vi "诊断标定3 - 副本.vi"(8 "CAN端口":u16(ring), 9 "设备索引号":u16(ring), 10 "CAN卡类型":u32(ring)=21) -> ()   [LabVIEW 2013] (continued)
                        n4271 = control-ref of="一级故障 2"() -> (w6031:refnum<vi>)
                        n4272 = property class="Clust (严格)"(reference=w6031) -> ("Value"=w6053:T10)  [unwired: 1 in, 2 out]
                        n4273 = Unbundle(w6053) -> ("总电压过高"=w6052:dbl, "整组电压不均衡"=w6047:dbl, "SOC过高"=w6040:dbl, "单体电压过高"=w6043:dbl, "总电压过低"=w6051:dbl, "温度过高"=w6050:dbl, "温度过低"=w6049:dbl, "单组电压不均衡"=w6048:dbl, "整组温度不均衡"=w6045:dbl, "单组温度不均衡"=w6046:dbl, "单体电压过低"=w6044:dbl, "充电电流过高"=w6042:dbl, "放电电流过高"=w6041:dbl, "SOC过低"=w6039:dbl, "内阻过大"=w6038:dbl, "极柱温度过高"=w6037:dbl, "SOH过低"=w6036:dbl)
                        n4274 = Build Array(w6052, w6051, w6050, w6049, w6048, w6047, w6046, w6045, w6043, w6044, w6042, w6041, w6040, w6039, w6038, w6037, w6036) -> (w6035:dbl[])
                        n4275 = for {
                          tunnel: w6035 -> [w6055] mode=indexing
                          tunnel: [w6054] -> w6034 mode=indexing
                          n4276 = Format Into String(format string="%#f" ("格式字符串"), w6055) -> (resulting string=w6054:string)  [unwired: 2 in, 1 out]
                        }
                        n4277 = Build Array(string[] ["总电压过高二级", "总电压过低二级", "温度过高二级", "温度过低二级", "单组电压不均衡二级", "整组电压不均衡二级", "单组温度不均衡二级", "整组温度不均衡二级", "单体电压过高二级", "单体电压过低二级", "充电电流过高二级", "放电电流过高二级", "SOC过高二级", "SOC过低二级", "内阻过大二级", "极柱温度过高二级", "SOH过低二级"], w6034) -> (w6032:string[][])
                        n4278 = Transpose 2D Array(2D array=w6032) -> (transposed array=w6030:string[][])
                      }
                      frame #3 {
                        n4279 = control-ref of="一级故障 3"() -> (w6058:refnum<vi>)
                        n4280 = property class="Clust (严格)"(reference=w6058) -> ("Value"=w6080:T10)  [unwired: 1 in, 2 out]
                        n4281 = Unbundle(w6080) -> ("总电压过高"=w6079:dbl, "整组电压不均衡"=w6074:dbl, "SOC过高"=w6067:dbl, "单体电压过高"=w6070:dbl, "总电压过低"=w6078:dbl, "温度过高"=w6077:dbl, "温度过低"=w6076:dbl, "单组电压不均衡"=w6075:dbl, "整组温度不均衡"=w6072:dbl, "单组温度不均衡"=w6073:dbl, "单体电压过低"=w6071:dbl, "充电电流过高"=w6069:dbl, "放电电流过高"=w6068:dbl, "SOC过低"=w6066:dbl, "内阻过大"=w6065:dbl, "极柱温度过高"=w6064:dbl, "SOH过低"=w6063:dbl)
                        n4282 = Build Array(w6079, w6078, w6077, w6076, w6075, w6074, w6073, w6072, w6070, w6071, w6069, w6068, w6067, w6066, w6065, w6064, w6063) -> (w6062:dbl[])
                        n4283 = for {
                          tunnel: w6062 -> [w6082] mode=indexing
                          tunnel: [w6081] -> w6061 mode=indexing
                          n4284 = Format Into String(format string="%#f" ("格式字符串"), w6082) -> (resulting string=w6081:string)  [unwired: 2 in, 1 out]
                        }
                        n4285 = Build Array(string[] ["总电压过高三级", "总电压过低三级", "温度过高三级", "温度过低三级", "单组电压不均衡三级", "整组电压不均衡三级", "单组温度不均衡三级", "整组温度不均衡三级", "单体电压过高三级", "单体电压过低三级", "充电电流过高三级", "放电电流过高三级", "SOC过高三级", "SOC过低三级", "内阻过大三级", "极柱温度过高三级", "SOH过低三级"], w6061) -> (w6059:string[][])
                        n4286 = Transpose 2D Array(2D array=w6059) -> (transposed array=w6057:string[][])
                      }
                      frame #4 {
                        n4287 = control-ref of="加热控制参数"() -> (w6095:refnum<vi>)
                        n4288 = property class="Clust (严格)"(reference=w6095) -> ("Value"=w6094:T11)  [unwired: 1 in, 2 out]
                        n4289 = Unbundle(w6094) -> ("风机开启温度"=w6093:dbl, "风机关闭温度"=w6092:dbl, "加热开启温度"=w6091:dbl, "加热关闭温度"=w6090:dbl, "风机开启温差"=w6089:dbl, "风机关闭温差"=w6088:dbl, "加热关闭温差"=w6084:dbl)
                        n4290 = Build Array(w6093, w6092, w6091, w6090, w6089, w6088, w6084) -> (w6087:dbl[])
                        n4291 = for {
                          tunnel: w6087 -> [w6097] mode=indexing
                          tunnel: [w6096] -> w6085 mode=indexing
                          n4292 = Format Into String(format string="%#f" ("格式字符串"), w6097) -> (resulting string=w6096:string)  [unwired: 2 in, 1 out]
                        }
                      }
                      frame #5 {
                        n4293 = control-ref of="充电控制参数"() -> (w6115:refnum<vi>)
                        n4294 = property class="Clust (严格)"(reference=w6115) -> ("Value"=w6117:T12)  [unwired: 1 in, 2 out]
                        n4295 = Unbundle(w6117) -> ("最大允许单体电压"=w6114:dbl, "最大允许总电压"=w6113:dbl, "最小允许单体电压"=w6112:dbl, "最大允许充电电流"=w6111:dbl, "最小允许充电电流"=w6110:dbl, "最大允许充电温度"=w6109:dbl, "最小允许充电温度"=w6108:dbl, "电流步长"=w6107:dbl)
                        n4296 = Build Array(w6114, w6113, w6112, w6111, w6110, w6109, w6108, w6107) -> (w6116:dbl[])
                        n4297 = for {
                          tunnel: w6116 -> [w6119] mode=indexing
                          tunnel: [w6118] -> w6101 mode=indexing
                          n4298 = Format Into String(format string="%#f" ("格式字符串"), w6119) -> (resulting string=w6118:string)  [unwired: 2 in, 1 out]
                        }
                        n4299 = Insert Into Array(array=w6102, new element=w6101) -> (w6100:string[])  [unwired: 1 in]
                        n4300 = Insert Into Array(array=w6104, new element=string[] ["最大允许单体电压", "最大允许总电压", "最小允许单体电压", "最大允许充电电流", "最小允许充电电流", "最大允许充电温度", "最小允许充电温度", "电流步长"]) -> (w6099:string[])  [unwired: 1 in]
                        n4301 = Build Array(w6099, w6100) -> (w6106:string[][])
                        n4302 = Transpose 2D Array(2D array=w6106) -> (transposed array=w6105:string[][])
                      }
                      frame #6 {
                        n4303 = control-ref of="电池信息"() -> (w6143:refnum<vi>)
                        n4304 = property class="Clust (严格)"(reference=w6143) -> ("Value"=w6146:T13)  [unwired: 1 in, 2 out]
                        n4305 = Unbundle(w6146) -> ("电池串联"=w6142:dbl, "电池并联"=w6141:dbl, "累计放电总安时"=w6139:dbl, "电池包额定容量"=w6138:dbl, "电池包额定能量(kWh)"=w6137:dbl, "电池包额定总电压"=w6136:dbl, "累计充电总安时"=w6140:dbl, "电池充满次数"=w6135:dbl, "电池放空次数"=w6134:dbl, "电池充电次数"=w6133:dbl, "电池生产日期"=w6131:string, "电池厂家"=w6130:string, "电池类型"=w6129:string, "电池包组号"=w6128:string, "电池包产权标识"=w6127:string, "电池应用车型"=w6126:string, "实际容量"=w6121:dbl)
                        n4306 = Build Array(w6131, w6130, w6129, w6128, w6127, w6126) -> (w6125:string[])
                        n4307 = Build Array(w6142, w6141, w6140, w6139, w6138, w6137, w6136, w6135, w6134, w6133, w6121) -> (w6132:dbl[])
                        n4308 = for {
                          tunnel: w6132 -> [w6148] mode=indexing
                          tunnel: [w6147] -> w6124 mode=indexing
                          n4309 = Format Into String(format string="%#f" ("格式字符串"), w6148) -> (resulting string=w6147:string)  [unwired: 2 in, 1 out]
                        }
                        n4310 = Insert Into Array(array=w6125, new element=w6124) -> (w6123:string[])  [unwired: 1 in]
                        n4311 = call <vilib>:"Unset Busy.vi"() -> ()  [unwired: 2 in, 10 out]
                        n4312 = Build Array(string[] ["电池生产日期", "电池厂商", "电池类型", "电池包组号", "电池包产权标识", "电池包应用车型", "电池串联", "电池并联", "累计充电总安时", "累计放电总安时", "电池包额定容量", "电池包额定能量", "电池包额定总电压", "电池充满次数", "电池放空次数", "电池充电次数", "实际容量"], w6123) -> (w6144:string[][])
                        n4313 = Transpose 2D Array(2D array=w6144) -> (transposed array=w6122:string[][])
                      }
                    }
                    n4314 = Insert Into Array(array=w5963, index (col)=2 ("禁用的索引 (列)"), new element #1=w5960, new element #2=w5959, new element #3=w5958, new element #4=w5957, new element #5=w5956) -> (w5961:string[][])  [unwired: 1 in]
                  }
                  frame "从板" {
                    n4315 = local read "从板号"() -> (w6160:u8)
                    n4316 = Number To Decimal String(number=w6160) -> (decimal integer string=w6157:string)  [unwired: 1 out]
                    n4317 = Concatenate Strings("S", w6157) -> (w6158:string)
                    n4318 = Build Array("从板号" ("元素"), w6157) -> (w6155:string[])
                    n4319 = stacked-sequence {
                      seq-local: [string[] ["风机开启温度", "风机关闭温度", "加热开启温度", "加热关闭温度", "风机开启温差", "风机关闭温差", "加热关闭温差"] _ _ _ _ _] -> [_ _ _ w6229 _ _]
                      seq-local: [w6172 _ _ _ _ _] -> [_ _ _ w6225 _ _]
                      seq-local: [_ string[] ["电压过高一级", "电压过低一级", "温度过高一级", "温度过低一级", "电压不均衡一级", "温度不均衡一级", "SOC过低一级"] _ _ _ _] -> [_ _ _ w6228 _ _]
                      seq-local: [_ w6190 _ _ _ _] -> [_ _ _ w6224 _ _]
                      seq-local: [_ _ string[] ["电压过高二级", "电压过低二级", "温度过高二级", "温度过低二级", "电压不均衡二级", "温度不均衡二级", "SOC过低二级"] _ _ _] -> [_ _ _ w6227 _ _]
                      seq-local: [_ _ w6205 _ _ _] -> [_ _ _ w6223 _ _]
                      tunnel: w6155 -> [w6185 _ _ _ _ _]
                      tunnel: [w6174 _ _ _ _ _] -> w6153
                      tunnel: [_ _ _ w6230 _ _] -> w6151
                      tunnel: [_ _ _ _ w6268 _] -> w6150
                      tunnel: [_ _ _ _ _ w6304] -> _
                      frame #0 {
                        w6165 = string[] ["", "", "", "", "", "", "", "", "", "", "  "]
                        n4320 = control-ref of="项目信息 2"() -> (w6184:refnum<vi>)
                        n4321 = property class="Tbl (严格)"(reference=w6184) -> ("Value"=w6162:string[][])  [unwired: 1 in, 2 out]
                        n4322 = control-ref of="加热控制参数"() -> (w6176:refnum<vi>)
                        n4323 = property class="Clust (严格)"(reference=w6176) -> ("Value"=w6183:T11)  [unwired: 1 in, 2 out]
                        n4324 = Unbundle(w6183) -> ("风机开启温度"=w6182:dbl, "风机关闭温度"=w6181:dbl, "加热开启温度"=w6180:dbl, "加热关闭温度"=w6179:dbl, "风机开启温差"=w6178:dbl, "风机关闭温差"=w6177:dbl, "加热关闭温差"=w6171:dbl)
                        n4325 = Build Array(w6182, w6181, w6180, w6179, w6178, w6177, w6171) -> (w6175:dbl[])
                        n4326 = for {
                          tunnel: w6175 -> [w6188] mode=indexing
                          tunnel: [w6187] -> w6172 mode=indexing
                          n4327 = Format Into String(format string="%#f" ("格式字符串"), w6188) -> (resulting string=w6187:string)  [unwired: 2 in, 1 out]
                        }
                        n4328 = Index Array(array=w6162, index (col)=0 ("禁用的索引 (列)")) -> (element=w6169:string[])  [unwired: 1 in]
                        n4329 = Index Array(array=w6162, index (col)=1 ("禁用的索引 (列)")) -> (element=w6168:string[])  [unwired: 1 in]
                        n4330 = Insert Into Array(array=w6169, new element=w6165) -> (w6167:string[])  [unwired: 1 in]
                        n4331 = Insert Into Array(array=w6168, new element=w6165) -> (w6166:string[])  [unwired: 1 in]
                        n4332 = Build Array(w6167, w6166) -> (w6163:string[][])
                        n4333 = Transpose 2D Array(2D array=w6163) -> (transposed array=w6161:string[][])
                        n4334 = Insert Into Array(array=w6161, index (row)=0 ("索引 (行)"), new element=w6185) -> (w6174:string[][])  [unwired: 1 in]
                      }
                      frame #1 {
                        n4335 = control-ref of="一级故障(从板)"() -> (w6201:refnum<vi>)
                        n4336 = property class="Clust (严格)"(reference=w6201) -> ("Value"=w6200:T15)  [unwired: 1 in, 2 out]
                        n4337 = Unbundle(w6200) -> ("电压过高"=w6199:dbl, "电压过低"=w6198:dbl, "温度过高"=w6197:dbl, "温度过低"=w6196:dbl, "电压不均衡(V)"=w6195:dbl, "温度不均衡"=w6194:dbl, "SOC过低"=w6193:dbl)
                        n4338 = Build Array(w6199, w6198, w6197, w6196, w6195, w6194, w6193) -> (w6192:dbl[])
                        n4339 = for {
                          tunnel: w6192 -> [w6203] mode=indexing
                          tunnel: [w6202] -> w6190 mode=indexing
                          n4340 = Format Into String(format string="%#f" ("格式字符串"), w6203) -> (resulting string=w6202:string)  [unwired: 2 in, 1 out]
                        }
                      }
                      frame #2 {
                        n4341 = control-ref of="二级故障(从板)"() -> (w6207:refnum<vi>)
                        n4342 = property class="Clust (严格)"(reference=w6207) -> ("Value"=w6216:T15)  [unwired: 1 in, 2 out]
                        n4343 = Unbundle(w6216) -> ("电压过高"=w6215:dbl, "电压过低"=w6214:dbl, "温度过高"=w6213:dbl, "温度过低"=w6212:dbl, "电压不均衡(V)"=w6211:dbl, "温度不均衡"=w6210:dbl, "SOC过低"=w6209:dbl)
                        n4344 = Build Array(w6215, w6214, w6213, w6212, w6211, w6210, w6209) -> (w6208:dbl[])
                        n4345 = for {
                          tunnel: w6208 -> [w6218] mode=indexing
                          tunnel: [w6217] -> w6205 mode=indexing
                          n4346 = Format Into String(format string="%#f" ("格式字符串"), w6218) -> (resulting string=w6217:string)  [unwired: 2 in, 1 out]
                        }
                      }
                      frame #3 {
                        n4347 = control-ref of="三级故障(从板)"() -> (w6231:refnum<vi>)
                        n4348 = property class="Clust (严格)"(reference=w6231) -> ("Value"=w6241:T15)  [unwired: 1 in, 2 out]
                        n4349 = Unbundle(w6241) -> ("电压过高"=w6240:dbl, "电压过低"=w6239:dbl, "温度过高"=w6238:dbl, "温度过低"=w6237:dbl, "电压不均衡(V)"=w6236:dbl, "温度不均衡"=w6235:dbl, "SOC过低"=w6234:dbl)
                        n4350 = Build Array(w6240, w6239, w6238, w6237, w6236, w6235, w6234) -> (w6233:dbl[])
                        n4351 = for {
                          tunnel: w6233 -> [w6243] mode=indexing
                          tunnel: [w6242] -> w6222 mode=indexing
                          n4352 = Format Into String(format string="%#f" ("格式字符串"), w6243) -> (resulting string=w6242:string)  [unwired: 2 in, 1 out]
                        }
                        n4353 = Insert Into Array(array=w6229, new element #1=w6228, new element #2=w6227, new element #3=string[] ["电压过高三级", "电压过低三级", "温度过高三级", "温度过低三级", "电压不均衡三级", "温度不均衡三级", "SOC过低三级"]) -> (w6220:string[])  [unwired: 1 in]
                        n4354 = Insert Into Array(array=w6225, new element #1=w6224, new element #2=w6223, new element #3=w6222) -> (w6221:string[])  [unwired: 1 in]
                        n4355 = Build Array(w6220, w6221) -> (w6232:string[][])
                        n4356 = Transpose 2D Array(2D array=w6232) -> (transposed array=w6230:string[][])
                      }
                      frame #4 {
                        n4357 = control-ref of="快换(从板)"() -> (w6267:refnum<vi>)
                        n4358 = property class="Clust (严格)"(reference=w6267) -> ("Value"=w6280:T16)  [unwired: 1 in, 2 out]
                        n4359 = Unbundle(w6280) -> ("串联数"=w6279:dbl, "并联数"=w6278:dbl, "电池厂家"=w6277:dbl, "电池类型"=w6276:dbl, "额定能量"=w6275:dbl, "额定容量"=w6274:dbl, "实际容量"=w6273:dbl, "额定总压"=w6266:dbl, "产权标识"=w6265:dbl, "应用车型"=w6264:dbl, "电池包组号"=w6263:dbl, "SOC"=w6261:dbl, "充电总安时"=w6260:dbl, "放电总安时"=w6259:dbl, "放空次数"=w6258:dbl, "充满次数"=w6257:dbl, "充电次数"=w6256:dbl, "车牌号"=w6246:string, "生产日期"=w6245:string, "最大允许单体电压"=w6255:dbl, "最大允许总电压"=w6254:dbl, "最大允许温度"=w6253:dbl, "最小允许温度"=w6252:dbl, "最大允许充电电流"=w6251:dbl, "最小允许充电电流"=w6250:dbl, "最小允许单体电压"=w6249:dbl, "电流步长"=w6248:dbl, "电池包序号"=w6247:dbl)
                        n4360 = Build Array(w6279, w6278, w6277, w6276, w6275, w6274, w6273, w6266, w6265, w6264, w6263, w6261, w6260, w6259, w6258, w6257, w6256, w6255, w6254, w6253, w6252, w6251, w6250, w6249, w6248, w6247) -> (w6272:dbl[])
                        n4361 = for {
                          tunnel: w6272 -> [w6282] mode=indexing
                          tunnel: [w6281] -> w6270 mode=indexing
                          n4362 = Format Into String(format string="%#f" ("格式字符串"), w6282) -> (resulting string=w6281:string)  [unwired: 2 in, 1 out]
                        }
                        n4363 = Insert Into Array(array=w6270, new element #1=w6246, new element #2=w6245) -> (w6262:string[])  [unwired: 1 in]
                        n4364 = call <vilib>:"Unset Busy.vi"() -> ()  [unwired: 2 in, 10 out]
                        n4365 = Build Array(string[] ["电池串联数", "电池并联数", "电池厂家", "额定能量", "额定容量", "实际容量", "额定总压", "产权标识", "应用车型", "电池包组号", "SOC", "充电总安时", "放电总安时", "放空次数", "充满次数", "充电次数", "最大允许单体电压", "最大允许总电压", "最大允许温度", "最小允许温度", "最大允许充电电流", "最小允许充电电流", "最小允许单体电压", "电流步长", "电池包序号"], w6262) -> (w6271:string[][])
                        n4366 = Transpose 2D Array(2D array=w6271) -> (transposed array=w6268:string[][])
                      }
                      frame #5 {
                        n4367 = local read "均衡参数"() -> (w6303:T17)
                        n4368 = Unbundle(w6303) -> ("充电结束电压(90%)"=w6295:sgl, "充电结束电压(91%)"=w6294:sgl, "充电结束电压(92%)"=w6293:sgl, "充电结束电压(93%)"=w6292:sgl, "充电结束电压(94%)"=w6291:sgl, "均衡计算-电压高阀值1级"=w6302:sgl, "均衡计算-电压高阀值2级"=w6301:sgl, "均衡计算-电压低阀值1级"=w6300:sgl, "均衡计算-电压低阀值2级"=w6299:sgl, "均衡计算-最低电压阀值"=w6298:sgl, "均衡停止-最低电压阀值"=w6297:sgl, "均衡计算-电压极差阀值"=w6296:sgl, "充电结束电压(95%)"=w6290:sgl, "充电结束电压(96%)"=w6289:sgl, "充电结束电压(97%)"=w6288:sgl, "充电结束电压(98%)"=w6287:sgl, "充电结束电压(99%)"=w6286:sgl, "充电结束电压(100%)"=w6285:sgl)
                        n4369 = Build Array(w6302, w6301, w6300, w6299, w6298, w6297, w6296, w6295, w6294, w6293, w6292, w6291, w6290, w6289, w6288, w6287, w6286, w6285) -> (w6307:sgl[])
                        n4370 = for {
                          tunnel: w6307 -> [w6309] mode=indexing
                          tunnel: [w6308] -> w6284 mode=indexing
                          n4371 = Format Into String(format string="%#f" ("格式字符串"), w6309) -> (resulting string=w6308:string)  [unwired: 2 in, 1 out]
                        }
                        n4372 = call <vilib>:"Unset Busy.vi"() -> ()  [unwired: 2 in, 10 out]
                        n4373 = Build Array(string[] ["均衡计算-电压高阀值1级", "均衡计算-电压高阀值2级", "均衡计算-电压低阀值1级", "均衡计算-电压低阀值2级", "均衡计算-最低电压阀值", "均衡停止-最低电压阀值", "均衡计算-电压极差阀值", "充电结束电压(90%)", "充电结束电压(91%)", "充电结束电压(92%)", "充电结束电压(93%)", "充电结束电压(94%)", "充电结束电压(95%)", "充电结束电压(96%)", "充电结束电压(97%)", "充电结束电压(98%)", "充电结束电压(99%)", "充电结束电压(100%)"], w6284) -> (w6306:string[][])
                        n4374 = Transpose 2D Array(2D array=w6306) -> (transposed array=w6304:string[][])
                      }
                    }
                    n4375 = Insert Into Array(array=w6153, index (col)=2 ("禁用的索引 (列)"), new element #1=w6151, new element #2=w6150) -> (w6152:string[][])  [unwired: 1 in]
                  }
                }
                n4376 = call "当前时间解析-8.6.vi"() -> ("名称格式时间"=w5944:string)  [unwired: 1 in, 18 out]
                n4377 = Concatenate Strings(w5944, w5943, ".txt" ("字符串")) -> (w5941:string)
                n4378 = call "自适应屏幕分辨率.vi"() -> ()  [unwired: 16 in]
                n4379 = call "文件对话框2"("prompt"="选择保存的路径", "default name"=w5941, "pattern (all files)"="*.txt") -> ("selected path"=w5939:path, "cancelled"=w5938:bool, "error out"=w5937:errorcluster)  [unwired: 9 in, 1 out]
                n4380 = call <vilib>:"Clear Errors.vi"("error in (no error)"=w5937) -> ()  [unwired: 6 in, 1 out]
                n4381 = case shown="假" w5938 {
                  tunnel: w5945 -> [w5950 _]
                  tunnel: w5939 -> [w5946 _]
                  frame False {
                    n4382 = call-poly <vilib>:"Write To Spreadsheet File.vi"("append to file? (new file:F)"=FALSE, "2D data"=w5950, "file path (dialog if empty)"=w5946) -> ("new file path (Not A Path if cancelled)"=w5948:path)  [unwired: 3 in, 2 out]
                    n4383 = Path To String(path=w5948) -> (string=w5947:string)
                    n4384 = stacked-sequence {
                      tunnel: w5947 -> [w5953]
                      frame #0 {
                        n4385 = Concatenate Strings("保存完成,路径为:" ("字符串"), w5953) -> (w5954:string)
                        n4386 = One Button Dialog(message=w5954, button name ("OK")="是" ("按钮名称（“确定”）")) -> ()  [unwired: 1 out]
                      }
                    }
                  }
                  frame True {
                  }
                }
              }
              frame Disabled {
                n4387 = stacked-sequence {
                  seq-local: [w6324] -> [_]
                  frame #0 {
                    n4388 = local read "项目信息"() -> (w6326:string[][])
                    n4389 = local read "项目信息2"() -> (w6323:T9)
                    n4390 = Array Subset(array=w6326, index (row)=0 ("索引"), index (col)=0 ("索引"), length (col)=2 ("索引")) -> (w6329:string[][])  [unwired: 1 in]
                    n4391 = local read "一级故障"() -> ()  [unwired: 1 out]
                    n4392 = local read "从板个数"() -> (w6324:dbl)
                    n4393 = Unbundle(w6323) -> ("电池额定容量(A)"=w6322:dbl, "电池实际容量(A)"=w6321:dbl, "车架(牌)号"=w6315:string, "配置文件版本"=w6314:string, "SOH(%)"=w6319:dbl, "SOC(%)"=w6320:dbl, "产品编号"=w6316:string)  [unwired: 2 out]
                    n4394 = Index Array(array=w6329, index (col) #1=1 ("禁用的索引 (列)"), index (col) #2=0 ("索引 (列)")) -> (element #1=w6313:string[], element #2=w6312:string[])  [unwired: 2 in]
                    n4395 = Build Array(w6322, w6321, w6320, w6319) -> (w6318:dbl[])
                    n4396 = Number To Decimal String(number=w6324) -> ()  [unwired: 1 in, 1 out]
                    n4397 = for {
                      tunnel: w6318 -> [w6334] mode=indexing
                      tunnel: [w6333] -> w6317 mode=indexing
                      n4398 = Format Into String(format string="%#f" ("格式字符串"), w6334) -> (resulting string=w6333:string)  [unwired: 2 in, 1 out]
                    }
                    n4399 = Insert Into Array(array=w6317, new element #1=w6316, new element #2=w6315, new element #3=w6314, new element #4=w6313) -> ()  [unwired: 1 in, 1 out]
                    n4400 = Insert Into Array(array=string[] ["电池额定容量", "电池实际容量", "SOC", "SOH", "产品编号", "车架(牌)号", "配置文件版本"], new element=w6312) -> ()  [unwired: 1 in, 1 out]
                  }
                }
              }
            }
          }
          frame "读配置文件" {
            n4401 = local read "主从选择"() -> (w6347:enum32{"主板", "从板"})
            n4402 = case shown="\"主板\", 默认" w6347 {
              tunnel: ["M" ("pattern (all files)") "S" ("pattern (all files)")] -> _
              tunnel: ["主板" ("pattern (all files)") "从板" ("pattern (all files)")] -> w6346
              frame "主板", Default {
              }
              frame "从板" {
              }
            }
            n4403 = case shown="真" "布尔" {
              tunnel: [w6749 w6754] -> w6339
              tunnel: [FALSE ("cancelled") w6753] -> _
              tunnel: w6346 -> [_ w6752]
              frame False {
                n4404 = local read "路径"() -> (w6749:path)
              }
              frame True {
                n4405 = global read "配置文件全局.vi" "诊断标定读取地址"() -> (w6750:path)
                n4406 = call "文件对话框"("start path"=w6750, "prompt"="选择要读取的配置文件", "button label"=w6752) -> ("selected path"=w6754:path, "cancelled"=w6753:bool, "error out"=w6751:errorcluster)  [unwired: 4 in, 6 out]
                n4407 = call <vilib>:"Clear Errors.vi"("error in (no error)"=w6751) -> ()  [unwired: 7 out]
              }
            }
            n4408 = Strip Path(path=w6339) -> (stripped path=w6335:path, name=w6343:string)
            n4409 = Match Pattern(string=w6343, regular expression=".ini" ("正则表达式")) -> (offset past match=w6341:i32)  [unwired: 1 in, 3 out]
            n4410 = control-ref of="结果"() -> (w6345:refnum<vi>)
            n4411 = global write "配置文件全局.vi" "诊断标定读取地址"(w6335) -> ()
            n4412 = Not Equal?(x=w6341, y=-1) -> (x != y?=w6336:bool)
            n4413 = case shown="真" w6336 {
              tunnel: w6339 -> [_ w6356]
              tunnel: [_ w6365] -> w6337
              frame False {
              }
              frame True {
                w6368 = "MD5码" ("key")
                w6369 = "总信息" ("section")
                n4414 = Strip Path(path=w6356) -> (stripped path=w6354:path, name=w6353:string)
                n4415 = Match Pattern(string=w6353, regular expression=".ini" ("正则表达式")) -> (before substring=w6350:string, match substring=w6351:string)  [unwired: 1 in, 2 out]
                n4416 = Concatenate Strings(w6350, "-rc" ("字符串"), w6351) -> (w6349:string)
                n4417 = Build Path(base path=w6354, name or relative path=w6349) -> (appended path=w6355:path)
                n4418 = Copy(10:w6355, 11:w6356) -> (3:w6360:path)  [unwired: 3 in, 2 out]
                n4419 = call <vilib>:"Open Config Data.vi"("create file if necessary (T)"=FALSE, "configuration file path"=w6360) -> ("refnum"=w6371:T25)  [unwired: 7 in, 2 out]
                n4420 = call-poly <vilib>:"Read Key.vi"("section"=w6369, "key"=w6368, "refnum"=w6371) -> ("value"=w6366:string, "refnum out"=w6370:T25)  [unwired: 5 in, 2 out]
                n4421 = call-poly <vilib>:"Write Key.vi"("section"=w6369, "value"=w6368, "key"=w6368, "refnum"=w6370) -> ("error out"=w6364:errorcluster, "found?"=w6363:bool, "refnum out"=w6362:T25)  [unwired: 5 in]
                n4422 = call <vilib>:"Close Config Data.vi"("error in (no error)"=w6364, "write file if changed (T)"=w6363, "refnum"=w6362) -> ("error out"=w6361:errorcluster, "file path"=w6358:path)  [unwired: 7 in]
                n4423 = call <vilib>:"MD5Checksum File.vi"("error in (no error)"=w6361, "Path"=w6358) -> ("error out"=w6359:errorcluster, "MD5 message-digest"=w6367:string)  [unwired: 8 in]
                n4424 = Equal?(x=w6367, y=w6366) -> (x = y?=w6365:bool)
                n4425 = Delete(path (use dialog)=w6358, error in=w6359) -> (error out=w6357:errorcluster)  [unwired: 3 in, 2 out]
                n4426 = call <vilib>:"Clear Errors.vi"("error in (no error)"=w6357) -> ()  [unwired: 6 in, 1 out]
              }
            }
            n4427 = And(x=w6336, y=w6337) -> (x .and. y?=w6338:bool)
            n4428 = case shown="真" w6338 {
              tunnel: w6339 -> [_ w6389]
              tunnel: w6345 -> [w6375 w6388]
              tunnel: w6337 -> [w6374 _]
              tunnel: w6336 -> [w6373 _]
              frame False {
                n4429 = stacked-sequence {
                  tunnel: w6373 -> [w6377 _]
                  tunnel: w6375 -> [w6376 w6383]
                  tunnel: w6374 -> [_ w6382]
                  frame #0 {
                    n4430 = case shown="假" w6377 {
                      tunnel: w6376 -> [w6379 _]
                      frame False {
                        n4431 = Build Array("文件格式错误") -> (w6380:string[])
                        n4432 = call "表格编辑.vi"("新元素/子数组"=w6380, "活动单元格:单元格背景色"=u32 16711680, "MCListbox引用句柄"=w6379) -> ()  [unwired: 9 out]
                      }
                      frame True {
                      }
                    }
                  }
                  frame #1 {
                    n4433 = case shown="假" w6382 {
                      tunnel: w6383 -> [w6385 _]
                      frame False {
                        n4434 = Build Array("文件MD5码验证错误") -> (w6386:string[])
                        n4435 = call "表格编辑.vi"("新元素/子数组"=w6386, "活动单元格:单元格背景色"=u32 16711680, "MCListbox引用句柄"=w6385) -> ()  [unwired: 9 out]
                      }
                      frame True {
                      }
                    }
                  }
                }
                n4436 = call <vilib>:"Unset Busy.vi"() -> ()  [unwired: 11 in, 1 out]
              }
              frame True {
                n4437 = stacked-sequence {
                  seq-local: [w6394 _ _ _] -> [_ w6622 w6716 _]
                  seq-local: [w6392 _ _ _] -> [_ w6600 _ _]
                  tunnel: w6389 -> [w6390 _ _ _]
                  tunnel: w6388 -> [w6407 _ _ w6743]
                  frame #0 {
                    w6391 = string[][] []
                    w6404 = "总信息" ("section")
                    n4438 = local write "路径"(w6390) -> ()
                    n4439 = call <vilib>:"Open Config Data.vi"("create file if necessary (T)"=FALSE, "configuration file path"=w6390) -> ("error out"=w6395:errorcluster, "refnum"=w6394:T25)  [unwired: 7 in, 1 out]
                    n4440 = call <vilib>:"Get Key Names.vi"("section"=w6404, "error in (no error)"=w6395, "refnum"=w6394) -> ("key names"=w6403:string[], "refnum out"=w6405:T25)  [unwired: 5 in, 2 out]
                    n4441 = for {
                      tunnel: w6405 -> [w6411]
                      tunnel: w6404 -> [w6410]
                      tunnel: w6403 -> [w6409] mode=indexing
                      tunnel: [w6408] -> w6400 mode=indexing
                      n4442 = call-poly <vilib>:"Read Key.vi"("section"=w6410, "key"=w6409, "refnum"=w6411) -> ("value"=w6408:string)  [unwired: 5 in, 3 out]
                    }
                    n4443 = Index Array(array=w6400) -> (element #1=w6393:string, element #2=w6398:string)  [unwired: 2 in]
                    n4444 = Decimal String To Number(string=w6393) -> (number=w6392:i32)  [unwired: 2 in, 1 out]
                    n4445 = Concatenate Strings("正在读取" ("字符串"), w6398, "的配置文件" ("字符串")) -> (w6396:string)
                    n4446 = Build Array(w6396) -> (w6401:string[])
                    n4447 = call "表格编辑.vi"("新元素/子数组"=w6401, "活动单元格:单元格背景色"=u32 6618880, "MCListbox引用句柄"=w6407) -> ()  [unwired: 9 out]
                    n4448 = local write "项目信息"(w6391) -> ()
                    n4449 = local write "项目信息 2"(w6391) -> ()
                  }
                  frame #1 {
                    w6582 = 20 ("长度")
                    w6623 = "主板" ("section")
                    n4450 = call <vilib>:"Get Key Names.vi"("section"=w6623, "refnum"=w6622) -> ("key names"=w6424:string[], "refnum out"=w6624:T25)  [unwired: 6 in, 2 out]
                    n4451 = for {
                      tunnel: w6624 -> [w6636]
                      tunnel: w6623 -> [w6635]
                      tunnel: w6424 -> [w6634] mode=indexing
                      tunnel: [w6633] -> w6423 mode=indexing
                      n4452 = call-poly <vilib>:"Read Key.vi"("section"=w6635, "key"=w6634, "refnum"=w6636) -> ("value"=w6633:string)  [unwired: 5 in, 3 out]
                    }
                    n4453 = Search 1D Array(1D array=w6424, element="总电压过高一级" ("元素"), start index (0)=0 ("开始索引(0)")) -> (index of element=w6504:i32)
                    n4454 = Search 1D Array(1D array=w6424, element="风机开启温度" ("元素"), start index (0)=w6504) -> (index of element=w6495:i32)
                    n4455 = Search 1D Array(1D array=w6424, element="电池串联" ("元素"), start index (0)=w6495) -> (index of element=w6493:i32)
                    n4456 = Decrement(x=w6504) -> (x-1=w6621:i32)
                    n4457 = Array Subset(array=w6424, index=1 ("索引"), length=w6621) -> (w6469:string[])
                    n4458 = Array Subset(array=w6423, index=1 ("索引"), length=w6621) -> (w6466:string[])
                    n4459 = Delete From Array(array=w6466, length=7 ("长度"), index=0 ("索引")) -> (deleted portion=w6463:string[], array with subset deleted=w6413:string[])
                    n4460 = Delete From Array(array=w6469, length=7 ("长度"), index=0 ("索引")) -> (array with subset deleted=w6422:string[])  [unwired: 1 out]
                    n4461 = Search 1D Array(1D array=w6424, element="分流器型号" ("元素")) -> (index of element=w6427:i32)  [unwired: 1 in]
                    n4462 = Index Array(array=w6423, index=0 ("索引")) -> (element=w6597:string)
                    n4463 = Decimal String To Number(string=w6597) -> (number=w6414:i32)  [unwired: 2 in, 1 out]
                    n4464 = Search 1D Array(1D array=w6422, element="主板电池节数" ("元素")) -> (index of element=w6588:i32)  [unwired: 1 in]
                    n4465 = Search 1D Array(1D array=w6422, element="主板温度起始值" ("元素")) -> (index of element=w6585:i32)  [unwired: 1 in]
                    n4466 = Search 1D Array(1D array=w6422, element="第一个保险通道" ("元素")) -> (index of element=w6584:i32)  [unwired: 1 in]
                    n4467 = Search 1D Array(1D array=w6422, element="主板温度个数" ("元素")) -> (index of element=w6586:i32)  [unwired: 1 in]
                    n4468 = Search 1D Array(1D array=w6422, element="主板电压起始值" ("元素")) -> (index of element=w6587:i32)  [unwired: 1 in]
                    n4469 = Search 1D Array(1D array=w6422, element="第1通道电压个数" ("元素")) -> (index of element=w6583:i32)  [unwired: 1 in]
                    n4470 = Index Array(array=w6423, index=w6427) -> (element=w6426:string)
                    n4471 = for {
                      N: 4 -> [_]
                      tunnel: w6463 -> [w6632] mode=indexing
                      tunnel: [w6631] -> w6612 mode=indexing
                      n4472 = Fract/Exp String To Number(string=w6632) -> (number=w6631:dbl)  [unwired: 3 in, 1 out]
                    }
                    n4473 = Increment(x=w6414) -> (x+1=w6596:i32)
                    n4474 = Increment(x=w6414) -> (x+1=w6581:i32)
                    n4475 = Increment(x=w6414) -> (x+1=w6594:i32)
                    n4476 = Increment(x=w6414) -> (x+1=w6595:i32)
                    n4477 = global write "读配置文件全局.vi" "从板个数"(w6414) -> ()
                    n4478 = local write "从板个数"(w6414) -> ()
                    n4479 = Decimal String To Number(string=w6426) -> (number=w6425:i32)  [unwired: 2 in, 1 out]
                    n4480 = Index Array(array=w6463, index #1=4 ("索引"), index #2=5 ("索引"), index #3=6 ("索引")) -> (element #1=w6603:string, element #2=w6602:string, element #3=w6601:string)
                    n4481 = Index Array(array=w6612) -> (element #1=w6610:dbl, element #2=w6609:dbl, element #3=w6608:dbl, element #4=w6607:dbl)  [unwired: 4 in]
                    n4482 = global write "EV05全局变量1.vi" "分流器型号"(w6425) -> ()
                    n4483 = Array Subset(array=w6413, index=w6588, length=w6596) -> (w6580:string[])
                    n4484 = Array Subset(array=w6413, index=w6587, length=w6595) -> (w6578:string[])
                    n4485 = Array Subset(array=w6413, index=w6586, length=w6594) -> (w6577:string[])
                    n4486 = Array Subset(array=w6413, index=w6585, length=w6581) -> (w6576:string[])
                    n4487 = Array Subset(array=w6413, index=w6584, length=20 ("长度")) -> (w6575:string[])
                    n4488 = Array Subset(array=w6413, index=w6583, length=w6582) -> (w6579:string[])
                    n4489 = Multiply(x=w6414, y=2) -> (x*y=w6415:i32)
                    n4490 = control-ref of="项目信息2"() -> (w6615:refnum<vi>)
                    n4491 = Array Subset(array=w6413, index=0 ("索引"), length=w6415) -> (w6412:string[])
                    n4492 = Insert Into Array(array=w6580, new element #1=w6579, new element #2=w6578, new element #3=w6577, new element #4=w6576, new element #5=w6575) -> ()  [unwired: 1 in, 1 out]
                    n4493 = property class="Clust (严格)"(reference=w6615) -> (reference out=w6613:refnum<vi>, "Value"=w6614:T9)  [unwired: 1 in, 1 out]
                    n4494 = Multiply(x=w6414, y=2) -> (x*y=w6419:i32)
                    n4495 = Array Subset(array=w6422, index=w6588, length=w6581) -> (w6453:string[])
                    n4496 = Array Subset(array=w6422, index=w6587, length=w6581) -> (w6451:string[])
                    n4497 = Array Subset(array=w6422, index=w6586, length=w6581) -> (w6450:string[])
                    n4498 = Array Subset(array=w6422, index=w6585) -> (w6449:string[])  [unwired: 1 in]
                    n4499 = Array Subset(array=w6422, index=w6584, length=w6582) -> (w6448:string[])
                    n4500 = Array Subset(array=w6422, index=w6583, length=w6582) -> (w6452:string[])
                    n4501 = Array Subset(array=w6422, index=0 ("索引"), length=w6419) -> (w6418:string[])
                    n4502 = global write "读配置文件全局.vi" "表格输入"(w6412) -> ()
                    n4503 = Build Array(w6418, w6412) -> (w6574:string[][])
                    n4504 = Bundle(cluster=w6614, "电池额定容量(A)"=w6610, "使用者"=w6600, "电池实际容量(A)"=w6609, "车架(牌)号"=w6602, "配置文件版本"=w6601, "SOH(%)"=w6607, "SOC(%)"=w6608, "产品编号"=w6603) -> (w6440:T9)  [unwired: 1 in]
                    n4505 = Transpose 2D Array(2D array=w6574) -> (transposed array=w6441:string[][])
                    n4506 = Multiply(x=w6414, y=4) -> (x*y=w6445:i32)
                    n4507 = Insert Into Array(array=w6453, new element #1=w6452, new element #2=w6451, new element #3=w6450, new element #4=w6449, new element #5=w6448) -> (w6447:string[])  [unwired: 1 in]
                    n4508 = Add(x=w6445, y=44) -> (x+y=w6443:i32)
                    n4509 = local write "项目信息"(w6441) -> ()
                    n4510 = property class="Clust (严格)"(reference=w6613, "Value"=w6440) -> ()  [unwired: 1 in, 2 out]
                    n4511 = global write "读配置文件全局.vi" "项目信息"(w6440) -> ()
                    n4512 = Array Subset(array=w6423, index=w6493, length=15 ("长度")) -> (w6431:string[])
                    n4513 = Array Subset(array=w6447, index=0 ("索引"), length=w6443) -> ()  [unwired: 1 out]
                    n4514 = Array Subset(array=w6423, index=w6495, length=15 ("长度")) -> (w6500:string[])
                    n4515 = Delete From Array(array=w6431, length=4 ("长度"), index=6 ("索引")) -> (deleted portion=w6487:string[], array with subset deleted=w6486:string[])
                    n4516 = for {
                      tunnel: w6500 -> [w6628] mode=indexing
                      tunnel: [w6627] -> w6499 mode=indexing
                      n4517 = Fract/Exp String To Number(string=w6628) -> (number=w6627:dbl)  [unwired: 3 in, 1 out]
                    }
                    n4518 = for {
                      tunnel: w6486 -> [w6626] mode=indexing
                      tunnel: [w6625] -> w6485 mode=indexing
                      n4519 = Fract/Exp String To Number(string=w6626) -> (number=w6625:dbl)  [unwired: 3 in, 1 out]
                    }
                    n4520 = Array Subset(array=w6423, index=w6504, length=51 ("长度")) -> (w6573:string[])
                    n4521 = for {
                      tunnel: w6573 -> [w6630] mode=indexing
                      tunnel: [w6629] -> w6572 mode=indexing
                      n4522 = Fract/Exp String To Number(string=w6630) -> (number=w6629:dbl)  [unwired: 3 in, 1 out]
                    }
                    n4523 = Index Array(array=w6485) -> (element #1=w6480:dbl, element #2=w6479:dbl, element #3=w6478:dbl, element #4=w6477:dbl, element #5=w6476:dbl, element #6=w6475:dbl, element #7=w6474:dbl, element #8=w6473:dbl, element #9=w6472:dbl, element #10=w6471:dbl, element #11=w6470:dbl)  [unwired: 11 in]
                    n4524 = Delete From Array(array=w6499, length=7 ("长度"), index=0 ("索引")) -> (deleted portion=w6436:dbl[], array with subset deleted=w6497:dbl[])
                    n4525 = Delete From Array(array=w6572, length=17 ("长度"), index=0 ("索引")) -> (deleted portion=w6433:dbl[], array with subset deleted=w6569:dbl[])
                    n4526 = Array To Cluster(array=w6436) -> (cluster=w6498:T26)
                    n4527 = global write "读配置文件全局.vi" "加热控制参数"(w6436) -> ()
                    n4528 = Index Array(array=w6497) -> (element #1=w6461:dbl, element #2=w6460:dbl, element #3=w6459:dbl, element #4=w6458:dbl, element #5=w6457:dbl, element #6=w6456:dbl, element #7=w6455:dbl, element #8=w6454:dbl)  [unwired: 8 in]
                    n4529 = Delete From Array(array=w6569, length=17 ("长度"), index=0 ("索引")) -> (deleted portion=w6432:dbl[], array with subset deleted=w6429:dbl[])
                    n4530 = Index Array(array=w6487) -> (element #1=w6484:string, element #2=w6483:string, element #3=w6481:string, element #4=w6482:string)  [unwired: 4 in]
                    n4531 = local write "加热控制参数"(w6498) -> ()
                    n4532 = global write "读配置文件全局.vi" "一级故障"(w6433) -> ()
                    n4533 = local read "一级故障 5"() -> (w6462:T12)
                    n4534 = control-ref of="电池信息"() -> (w6491:refnum<vi>)
                    n4535 = global write "读配置文件全局.vi" "二级故障"(w6432) -> ()
                    n4536 = global write "读配置文件全局.vi" "三级故障"(w6429) -> ()
                    n4537 = Bundle(cluster=w6462, "最大允许单体电压"=w6461, "最大允许总电压"=w6457, "最小允许单体电压"=w6460, "最大允许充电电流"=w6459, "最小允许充电电流"=w6458, "最大允许充电温度"=w6456, "最小允许充电温度"=w6455, "电流步长"=w6454) -> (w6435:T12)
                    n4538 = property class="Clust (严格)"(reference=w6491) -> (reference out=w6492:refnum<vi>, "Value"=w6490:T13)  [unwired: 1 in, 1 out]
                    n4539 = Bundle(cluster=w6490, "电池串联"=w6480, "电池并联"=w6479, "累计放电总安时"=w6473, "电池包额定容量"=w6478, "电池包额定能量(kWh)"=w6477, "电池包额定总电压"=w6476, "累计充电总安时"=w6474, "电池充满次数"=w6471, "电池放空次数"=w6472, "电池充电次数"=w6470, "电池生产日期"=w6481, "电池厂家"=w6484, "电池类型"=w6483, "电池包组号"=w6482, "实际容量"=w6475) -> (w6430:T13)  [unwired: 2 in]
                    n4540 = Cluster To Array(cluster=w6435) -> (array=w6434:dbl[])
                    n4541 = local write "一级故障 5"(w6435) -> ()
                    n4542 = global write "读配置文件全局.vi" "充电控制参数"(w6434) -> ()
                    n4543 = Index Array(array=w6433) -> (element #1=w6562:dbl, element #2=w6561:dbl, element #3=w6560:dbl, element #4=w6559:dbl, element #5=w6558:dbl, element #6=w6557:dbl, element #7=w6556:dbl, element #8=w6555:dbl, element #9=w6554:dbl, element #10=w6553:dbl, element #11=w6552:dbl, element #12=w6551:dbl, element #13=w6550:dbl, element #14=w6549:dbl, element #15=w6548:dbl, element #16=w6547:dbl, element #17=w6546:dbl)  [unwired: 17 in]
                    n4544 = global write "读配置文件全局.vi" "电池信息"(w6430) -> ()
                    n4545 = Index Array(array=w6432) -> (element #1=w6529:dbl, element #2=w6530:dbl, element #3=w6531:dbl, element #4=w6532:dbl, element #5=w6533:dbl, element #6=w6534:dbl, element #7=w6535:dbl, element #8=w6536:dbl, element #9=w6537:dbl, element #10=w6538:dbl, element #11=w6539:dbl, element #12=w6540:dbl, element #13=w6541:dbl, element #14=w6542:dbl, element #15=w6543:dbl, element #16=w6544:dbl, element #17=w6545:dbl)  [unwired: 17 in]
                    n4546 = Index Array(array=w6429) -> (element #1=w6524:dbl, element #2=w6523:dbl, element #3=w6522:dbl, element #4=w6521:dbl, element #5=w6520:dbl, element #6=w6519:dbl, element #7=w6518:dbl, element #8=w6517:dbl, element #9=w6516:dbl, element #10=w6515:dbl, element #11=w6514:dbl, element #12=w6513:dbl, element #13=w6512:dbl, element #14=w6511:dbl, element #15=w6510:dbl, element #16=w6509:dbl, element #17=w6508:dbl)  [unwired: 17 in]
                    n4547 = control-ref of="一级故障 3"() -> (w6507:refnum<vi>)
                    n4548 = control-ref of="一级故障 2"() -> (w6526:refnum<vi>)
                    n4549 = property class="Clust (严格)"(reference=w6526) -> (reference out=w6528:refnum<vi>, "Value"=w6527:T10)  [unwired: 1 in, 1 out]
                    n4550 = property class="Clust (严格)"(reference=w6507) -> (reference out=w6506:refnum<vi>, "Value"=w6525:T10)  [unwired: 1 in, 1 out]
                    n4551 = property class="Clust (严格)"(reference=w6492, "Value"=w6430) -> ()  [unwired: 1 in, 2 out]
                    n4552 = Bundle(cluster=w6527, "总电压过高"=w6529, "整组电压不均衡"=w6533, "SOC过高"=w6541, "单体电压过高"=w6537, "总电压过低"=w6530, "温度过高"=w6531, "温度过低"=w6532, "单组电压不均衡"=w6534, "整组温度不均衡"=w6535, "单组温度不均衡"=w6536, "单体电压过低"=w6538, "充电电流过高"=w6539, "放电电流过高"=w6540, "SOC过低"=w6542, "内阻过大"=w6543, "极柱温度过高"=w6544, "SOH过低"=w6545) -> (w6438:T10)
                    n4553 = Bundle(cluster=w6525, "总电压过高"=w6524, "整组电压不均衡"=w6520, "SOC过高"=w6512, "单体电压过高"=w6516, "总电压过低"=w6523, "温度过高"=w6522, "温度过低"=w6521, "单组电压不均衡"=w6519, "整组温度不均衡"=w6518, "单组温度不均衡"=w6517, "单体电压过低"=w6515, "充电电流过高"=w6514, "放电电流过高"=w6513, "SOC过低"=w6511, "内阻过大"=w6510, "极柱温度过高"=w6509, "SOH过低"=w6508) -> (w6437:T10)
                    n4554 = control-ref of="一级故障"() -> (w6565:refnum<vi>)
                    n4555 = property class="Clust (严格)"(reference=w6565) -> (reference out=w6563:refnum<vi>, "Value"=w6564:T10)  [unwired: 1 in, 1 out]
                    n4556 = Bundle(cluster=w6564, "总电压过高"=w6562, "整组电压不均衡"=w6558, "SOC过高"=w6550, "单体电压过高"=w6554, "总电压过低"=w6561, "温度过高"=w6560, "温度过低"=w6559, "单组电压不均衡"=w6557, "整组温度不均衡"=w6556, "单组温度不均衡"=w6555, "单体电压过低"=w6553, "充电电流过高"=w6552, "放电电流过高"=w6551, "SOC过低"=w6549, "内阻过大"=w6548, "极柱温度过高"=w6547, "SOH过低"=w6546) -> (w6439:T10)
                    n4557 = property class="Clust (严格)"(reference=w6563, "Value"=w6439) -> ()  [unwired: 1 in, 2 out]
                    n4558 = property class="Clust (严格)"(reference=w6528, "Value"=w6438) -> ()  [unwired: 1 in, 2 out]
                    n4559 = property class="Clust (严格)"(reference=w6506, "Value"=w6437) -> ()  [unwired: 1 in, 2 out]
                  }
                  frame #2 {
                    w6701 = 1 ("索引")
                    # "均衡计算-电压高阀值1级"
                    n4560 = call <vilib>:"Get Section Names.vi"("refnum"=w6716) -> ("section names"=w6717:string[], "refnum out"=w6721:T25)  [unwired: 8 in, 1 out]
                    n4561 = local read "从板号"() -> (w6699:u8)
                    n4562 = Delete From Array(array=w6717, length=2 ("长度"), index=0 ("索引")) -> (array with subset deleted=w6720:string[])  [unwired: 1 out]
                    n4563 = for {
                      tunnel: w6720 -> [w6737] mode=indexing
                      tunnel: w6721 -> [w6738]
                      tunnel: [w6730] -> w6698 mode=indexing
                      tunnel: [w6729] -> w6642
                      n4564 = call <vilib>:"Get Key Names.vi"("section"=w6737, "refnum"=w6738) -> ("key names"=w6729:string[], "refnum out"=w6736:T25)  [unwired: 6 in, 2 out]
                      n4565 = for {
                        tunnel: w6729 -> [w6742] mode=indexing
                        tunnel: w6737 -> [w6741]
                        tunnel: w6736 -> [w6740]
                        tunnel: [w6739] -> w6730 mode=indexing
                        n4566 = call-poly <vilib>:"Read Key.vi"("section"=w6741, "key"=w6742, "refnum"=w6740) -> ("value"=w6739:string)  [unwired: 5 in, 3 out]
                      }
                      n4567 = Index Array(array=w6730, index=0 ("索引")) -> (element=w6733:string)
                      n4568 = local read "输出数组"() -> (w6734:string[][])
                      n4569 = Decimal String To Number(string=w6733) -> (number=w6732:i32)  [unwired: 2 in, 1 out]
                      n4570 = Decrement(x=w6732) -> (x-1=w6728:i32)
                      n4571 = Replace Array Subset(array=w6734, new element=w6730, index (col)=w6728) -> (w6731:string[][])  [unwired: 1 in]
                      n4572 = local write "输出数组"(w6731) -> ()
                    }
                    "key names" <- w6642
                    n4573 = Decrement(x=w6699) -> (x-1=w6715:u8)
                    n4574 = Index Array(array=w6698, index (row)=w6715) -> (element=w6641:string[])  [unwired: 1 in]
                    n4575 = Search 1D Array(1D array=w6642, element="风机开启温度" ("元素")) -> (index of element=w6704:i32)  [unwired: 1 in]
                    n4576 = Search 1D Array(1D array=w6642, element="电压过高一级" ("元素"), start index (0)=w6704) -> (index of element=w6667:i32)
                    n4577 = Search 1D Array(1D array=w6642, element="均衡计算-电压高阀值1级" ("元素"), start index (0)=w6667) -> (index of element=w6665:i32)
                    n4578 = Array Subset(array=w6641, index=w6665, length=17 ("长度")) -> (w6664:string[])
                    n4579 = Decrement(x=w6704) -> (x-1=w6702:i32)
                    n4580 = Array Subset(array=w6641, index=w6701, length=w6702) -> (w6639:string[])
                    n4581 = Array Subset(array=w6641, index=w6667, length=21 ("长度")) -> (w6713:string[])
                    n4582 = Array Subset(array=w6642, index=w6701, length=w6702) -> (w6678:string[])
                    n4583 = Index Array(array=w6641, index=0 ("索引")) -> (element=w6673:string)
                    n4584 = Array Subset(array=w6641, index=w6704, length=7 ("长度")) -> (w6707:string[])
                    n4585 = for {
                      tunnel: w6664 -> [w6723] mode=indexing
                      tunnel: [w6722] -> w6663 mode=indexing
                      n4586 = Fract/Exp String To Number(string=w6723) -> (number=w6722:dbl)  [unwired: 3 in, 1 out]
                    }
                    n4587 = for {
                      tunnel: w6713 -> [w6725] mode=indexing
                      tunnel: [w6724] -> w6714 mode=indexing
                      n4588 = Fract/Exp String To Number(string=w6725) -> (number=w6724:dbl)  [unwired: 3 in, 1 out]
                    }
                    n4589 = Decimal String To Number(string=w6673) -> (number=w6672:i32)  [unwired: 2 in, 1 out]
                    n4590 = for {
                      tunnel: w6707 -> [w6727] mode=indexing
                      tunnel: [w6726] -> w6675 mode=indexing
                      n4591 = Fract/Exp String To Number(string=w6727) -> (number=w6726:dbl)  [unwired: 3 in, 1 out]
                    }
                    n4592 = global write "读配置文件全局2.vi" "从板板号"(w6672) -> ()
                    n4593 = Delete From Array(array=w6714, length=7 ("长度"), index=0 ("索引")) -> (deleted portion=w6677:dbl[], array with subset deleted=w6710:dbl[])
                    n4594 = Array To Cluster(array=w6675) -> (cluster=w6697:T26)
                    n4595 = global write "读配置文件全局2.vi" "加热控制参数"(w6675) -> ()
                    n4596 = Delete From Array(array=w6710, length=7 ("长度"), index=0 ("索引")) -> (deleted portion=w6670:dbl[], array with subset deleted=w6671:dbl[])
                    n4597 = local write "加热控制参数"(w6697) -> ()
                    n4598 = Array To Cluster(array=w6677) -> (cluster=w6681:T26)
                    n4599 = Array To Cluster(array=w6671) -> (cluster=w6679:T26)
                    n4600 = Array To Cluster(array=w6670) -> (cluster=w6680:T26)
                    n4601 = global write "读配置文件全局2.vi" "三级故障阀值"(w6671) -> ()
                    n4602 = global write "读配置文件全局2.vi" "一级故障阀值"(w6677) -> ()
                    n4603 = global write "读配置文件全局2.vi" "二级故障阀值"(w6670) -> ()
                    n4604 = local write "一级故障 6"(w6681) -> ()
                    n4605 = local write "一级故障 8"(w6679) -> ()
                    n4606 = local write "一级故障 7"(w6680) -> ()
                    n4607 = Search 1D Array(1D array=w6678, element="第1通道电压个数" ("元素")) -> (index of element=w6689:i32)  [unwired: 1 in]
                    n4608 = Search 1D Array(1D array=w6678, element="电压个数" ("元素")) -> ()  [unwired: 1 in, 1 out]
                    n4609 = Search 1D Array(1D array=w6678, element="温度个数" ("元素")) -> (index of element=w6691:i32)  [unwired: 1 in]
                    n4610 = Search 1D Array(1D array=w6678, element="第一个保险通道" ("元素")) -> (index of element=w6690:i32)  [unwired: 1 in]
                    n4611 = Array Subset(array=w6639, length=2 ("长度")) -> (w6686:string[])  [unwired: 1 in]
                    n4612 = Array Subset(array=w6639, index=w6691, length=2 ("长度")) -> (w6684:string[])
                    n4613 = Array Subset(array=w6639, index=w6690, length=20 ("长度")) -> (w6683:string[])
                    n4614 = Array Subset(array=w6639, index=w6689, length=20 ("长度")) -> (w6685:string[])
                    n4615 = Array Subset(array=w6639, length=27 ("长度")) -> (w6638:string[])  [unwired: 1 in]
                    n4616 = Insert Into Array(array=w6686, new element #1=w6685, new element #2=w6684, new element #3=w6683) -> ()  [unwired: 1 in, 1 out]
                    n4617 = Build Array(string[] ["电压个数", "温度个数", "第一个保险通道", "第一个保险位置", "第二个保险通道", "第二个保险位置", "第三个保险通道", "第三个保险位置", "第四个保险通道", "第四个保险位置", "第五个保险通道", "第五个保险位置", "第六个保险通道", "第六个保险位置", "第七个保险通道", "第七个保险位置", "第八个保险通道", "第八个保险位置", "第九个保险通道", "第九个保险位置", "第十个保险通道", "第十个保险位置", "第1通道电压个数", "第2通道电压个数", "第3通道电压个数", "第4通道电压个数", "第5通道电压个数"], w6638) -> (w6682:string[][])
                    n4618 = global write "读配置文件全局2.vi" "表格"(w6638) -> ()
                    n4619 = Index Array(array=w6663) -> (element #1=w6660:dbl, element #2=w6659:dbl, element #3=w6658:dbl, element #4=w6657:dbl, element #5=w6656:dbl, element #6=w6655:dbl, element #7=w6654:dbl, element #8=w6653:dbl, element #9=w6652:dbl, element #10=w6651:dbl, element #11=w6650:dbl, element #12=w6649:dbl, element #13=w6648:dbl, element #14=w6647:dbl, element #15=w6646:dbl, element #16=w6645:dbl, element #17=w6644:dbl, element #18=w6643:dbl)  [unwired: 18 in]
                    n4620 = Transpose 2D Array(2D array=w6682) -> (transposed array=w6676:string[][])
                    n4621 = local write "项目信息 2"(w6676) -> ()
                    n4622 = local read "均衡参数"() -> (w6662:T17)
                    n4623 = Bundle(cluster=w6662, "充电结束电压(90%)"=w6653, "充电结束电压(91%)"=w6652, "充电结束电压(92%)"=w6651, "充电结束电压(93%)"=w6650, "充电结束电压(94%)"=w6649, "均衡计算-电压高阀值1级"=w6660, "均衡计算-电压高阀值2级"=w6659, "均衡计算-电压低阀值1级"=w6658, "均衡计算-电压低阀值2级"=w6657, "均衡计算-最低电压阀值"=w6656, "均衡停止-最低电压阀值"=w6655, "均衡计算-电压极差阀值"=w6654, "充电结束电压(95%)"=w6648, "充电结束电压(96%)"=w6647, "充电结束电压(97%)"=w6646, "充电结束电压(98%)"=w6645, "充电结束电压(99%)"=w6644, "充电结束电压(100%)"=w6643) -> (w6661:T17)
                    n4624 = local write "均衡参数"(w6661) -> ()
                  }
                  frame #3 {
                    n4625 = call <vilib>:"Unset Busy.vi"() -> ()  [unwired: 11 in, 1 out]
                    n4626 = Build Array("读取完成") -> (w6746:string[])
                    n4627 = property on="全部写入" class="Bool (严格)"("DisabledEnum"=0) -> ()  [unwired: 2 in, 2 out]
                    n4628 = call "表格编辑.vi"("新元素/子数组"=w6746, "活动单元格:单元格背景色"=u32 6618880, "MCListbox引用句柄"=w6743) -> ()  [unwired: 9 out]
                  }
                }
              }
            }
          }
        }
      }
      frame Error {
      }
    }
  }
  n4629 = Release Queue(queue=w28, force destroy? (F)=TRUE ("强制销毁？(F)"), error in (no error)=w27) -> (error out=w30:errorcluster)  [unwired: 2 out]
  n4630 = call <vilib>:"Clear Errors.vi"("error in (no error)"=w30) -> ()  [unwired: 7 out]
  n4631 = local write "面板选择"(T7."读写参数" ("面板选择")) -> ()
  n4632 = Release Queue(queue=w34, force destroy? (F)=TRUE ("强制销毁？(F)"), error in (no error)=w33) -> (error out=w31:errorcluster)  [unwired: 2 out]
  n4633 = call <vilib>:"Clear Errors.vi"("error in (no error)"=w31) -> ()  [unwired: 7 out]
